vi "LV4_2.vi"() -> ()   [LabVIEW 2011]
uses:
  <vilib>/imath/engines/lvmath2/RunTimeEngine/ErrorHandling/NIMS_Finalize Error.vi
  <vilib>/imath/engines/lvmath2/RunTimeEngine/NodeEndStatement/NIMS_NodeEndStatement_Output.vi
  <instcachedir>/0/NIMS_NodeEndStatement_Output_53EC0D466D134D7ABD903AC30B43404B.lvgen/NIMS_NodeEndStatement_Output_53EC0D466D134D7ABD903AC30B43404B_002.vi
  <instcachedir>/0/NIMS_NodeEndStatement_Output_53EC0D466D134D7ABD903AC30B43404B.lvgen/NIMS_NodeEndStatement_Output_53EC0D466D134D7ABD903AC30B43404B_005.vi
  <instcachedir>/0/NIMS_NodeEndStatement_Output_53EC0D466D134D7ABD903AC30B43404B.lvgen/NIMS_NodeEndStatement_Output_53EC0D466D134D7ABD903AC30B43404B_003.vi
  <vilib>/imath/engines/lvmath2/RunTimeEngine/BuiltInFunctions/linramp/NIMS_linramp.vi
  <vilib>/imath/engines/lvmath2/RunTimeEngine/BuiltInFunctions/residue/NIMS_residue_To Partial Fraction Expansion.vi
  <vilib>/imath/engines/lvmath2/RunTimeEngine/ErrorHandling/NIMS_Error From Error Code.vi
  <vilib>/imath/engines/lvmath2/RunTimeEngine/ArithmeticOperatorToken/NIMS_ArithmeticOperator_multmx.vi
  <instcachedir>/0/NIMS_ArithmeticOperator_multmx_7C179C1E3F6A47AEB223A71AB1A54D0B.lvgen/NIMS_ArithmeticOperator_multmx_7C179C1E3F6A47AEB223A71AB1A54D0B_006.vi
  <vilib>/imath/engines/lvmath2/RunTimeEngine/ArithmeticOperatorToken/NIMS_ArithmeticOperator_multmx(RV,M).vi
  <instcachedir>/0/NIMS_ArithmeticOperator_multmx(RV,M)_0F69384DF375434AAFCFC7849B80E797.lvgen/NIMS_ArithmeticOperator_multmx(RV,M)_0F69384DF375434AAFCFC7849B80E797_000.vi
  <vilib>/imath/engines/lvmath2/RunTimeEngine/ErrorHandling/NIMS_Create Error From Enums.vi
  <vilib>/imath/engines/lvmath2/RunTimeEngine/VariableToken/Read/NIMS_Get Elements - CV(_) - Check.vi
  <instcachedir>/0/NIMS_Get Elements - CV(_) - Check_4CF014B95B49446692066C44E7C19A08.lvgen/NIMS_Get Elements - CV(_) - Check_4CF014B95B49446692066C44E7C19A08_001.vi
  <vilib>/imath/engines/lvmath2/RunTimeEngine/ArithmeticOperatorToken/NIMS_ArithmeticOperator_times.vi
  <instcachedir>/0/NIMS_ArithmeticOperator_times_3FA9DDB491BD45F6905798C0465C9825.lvgen/NIMS_ArithmeticOperator_times_3FA9DDB491BD45F6905798C0465C9825_003.vi
  <vilib>/imath/engines/lvmath2/RunTimeEngine/ArithmeticOperatorToken/NIMS_ArithmeticOperator_plus.vi
  <instcachedir>/0/NIMS_ArithmeticOperator_plus_1E95F7DAB906458CBECCADBE8E6FD739.lvgen/NIMS_ArithmeticOperator_plus_1E95F7DAB906458CBECCADBE8E6FD739_001.vi
  <vilib>/imath/engines/lvmath2/RunTimeEngine/BuiltInFunctions/conv/NIMS_conv(V,V).vi
  <instcachedir>/0/NIMS_conv(V,V)_D3E194F2B5174935BB2368CEB7AAC5A9.lvgen/NIMS_conv(V,V)_D3E194F2B5174935BB2368CEB7AAC5A9_000.vi
  <instcachedir>/0/NIMS_Get Elements - CV(_) - Check_4CF014B95B49446692066C44E7C19A08.lvgen/NIMS_Get Elements - CV(_) - Check_4CF014B95B49446692066C44E7C19A08_002.vi
  <instcachedir>/0/NIMS_ArithmeticOperator_times_3FA9DDB491BD45F6905798C0465C9825.lvgen/NIMS_ArithmeticOperator_times_3FA9DDB491BD45F6905798C0465C9825_008.vi
  <instcachedir>/0/NIMS_ArithmeticOperator_plus_1E95F7DAB906458CBECCADBE8E6FD739.lvgen/NIMS_ArithmeticOperator_plus_1E95F7DAB906458CBECCADBE8E6FD739_009.vi
panel:
  out "Cosine Response":cluster{"t":dbl[], "xstep2":dbl[]}[](graph)
  out "Ramp Response":cluster{"t":dbl[], "xstep2":dbl[]}[](graph)
  out "Step Response":cluster{"t":dbl[], "xstep2":dbl[]}[](graph)
  in  "Period":dbl(slide)=1.0 scale=0.5..5.0
  in  "K2":dbl(slide)=2.0 scale=0.0..10.0
  in  "K1":dbl(slide)=1.25 scale=0.7..2.0
  in  "stop":bool
  in  "K":dbl(slide)=1.25 scale=0.7..2.0
  # "L = 0.625 cm"
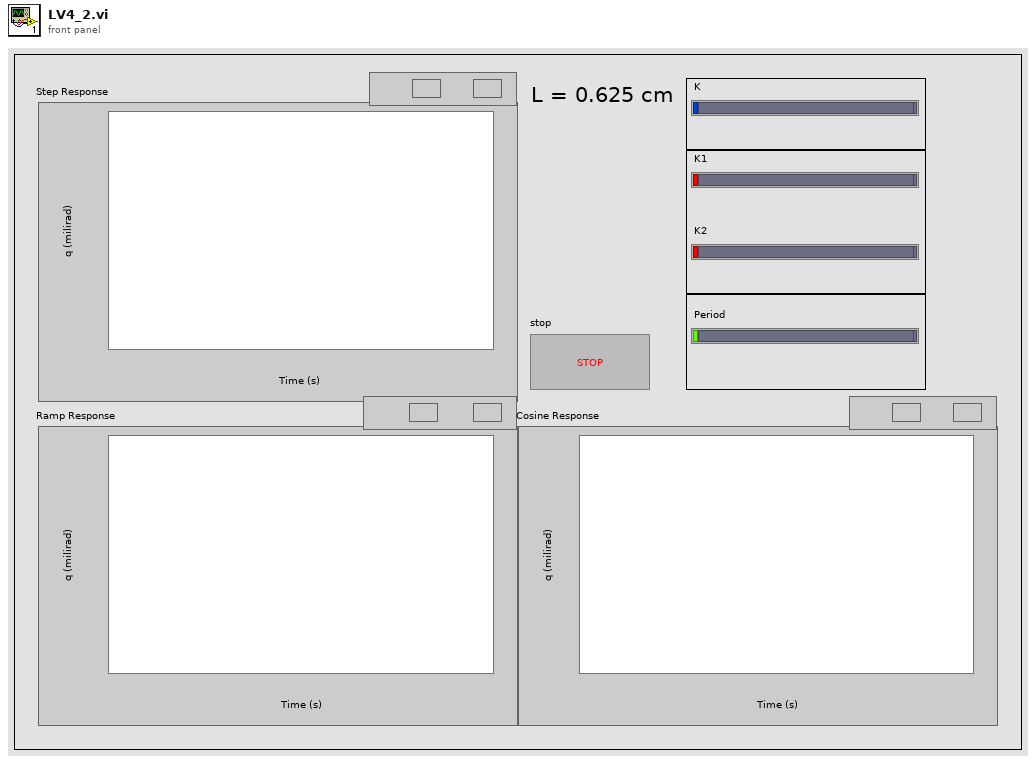
[diagram p1: front panel]
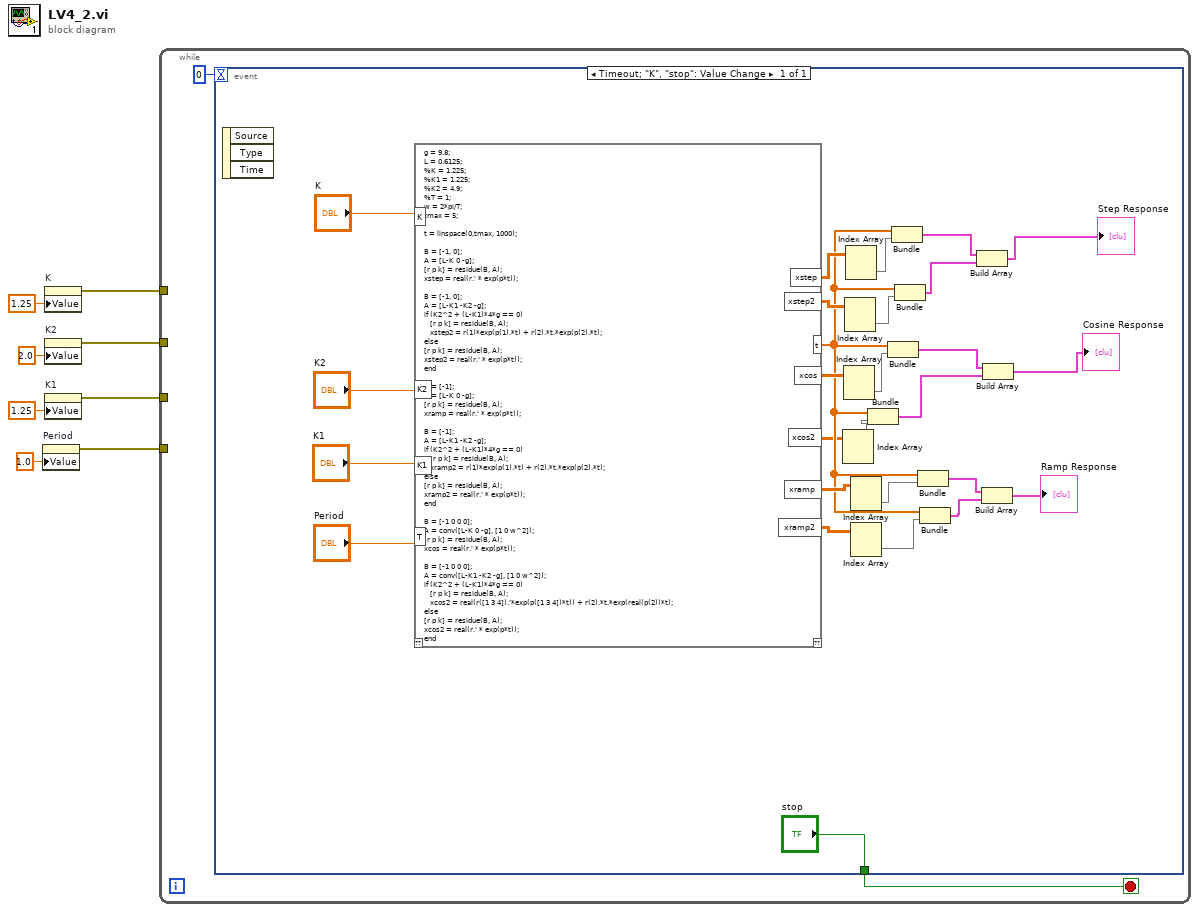
[diagram p0: block diagram]
diagram:
  n1 = property on="Period" class="Slide (strict)"("Value"=1.0 ("Period")) -> (error out=w5:errorcluster)  [unwired: 2 in, 1 out]
  n2 = property on="K" class="Slide (strict)"("Value"=1.25 ("K")) -> (error out=w8:errorcluster)  [unwired: 2 in, 1 out]
  n3 = property on="K2" class="Slide (strict)"("Value"=2.0 ("K2")) -> (error out=w7:errorcluster)  [unwired: 2 in, 1 out]
  n4 = property on="K1" class="Slide (strict)"("Value"=1.25 ("K1")) -> (error out=w6:errorcluster)  [unwired: 2 in, 1 out]
  n5 = while {
    tunnel: w8 -> [_]
    tunnel: w7 -> [_]
    tunnel: w6 -> [_]
    tunnel: w5 -> [_]
    stop <- w10 stop-if-true
    n6 = event shown="[0] Timeout;  \"K\", \"stop\": Value Change" {
      selector: _ -> [_]
      dyn-events: _ -> [_]
      timeout: 0 -> [_]
      tunnel: ["stop"] -> w10
      event Timeout; "K", "stop": Value Change {
        n7 = event-data() -> ()  [unwired: 1 in, 3 out]
        n8 = mathscript code="g = 9.8;\nL = 0.6125;\n%K = 1.225;\n%K1 = 1.225;\n%K2 = 4.9;\n%T = 1;\nw = 2*pi/T;\ntmax = 5;\n\nt = linspace(0,tmax, 1000);\n\nB = [-1, 0];\nA = [L-K 0 -g];\n[r p k] = residue(B, A);\nxstep = real(r.' * exp(p*t));\n\nB = [-1, 0];\nA = [L-K1 -K2 -g];\nif (K2^2 + (L-K1)*4*g == 0)\n   [r p k] = residue(B, A);\n   xstep2 = r(1)*exp(p(1).*t) + r(2).*t.*exp(p(2).*t);\nelse\n[r p k] = residue(B, A);\nxstep2 = real(r.' * exp(p*t));\nend\n\nB = [-1];\nA = [L-K 0 -g];\n[r p k] = residue(B, A);\nxramp = real(r.' * exp(p*t));\n\nB = [-1];\nA = [L-K1 -K2 -g];\nif (K2^2 + (L-K1)*4*g == 0)\n   [r p k] = residue(B, A);\n   xramp2 = r(1)*exp(p(1).*t) + r(2).*t.*exp(p(2).*t);\nelse\n[r p k] = residue(B, A);\nxramp2 = real(r.' * exp(p*t));\nend\n\nB = [-1 0 0 0];\nA = conv([L-K 0 -g], [1 0 w^2]);\n[r p k] = residue(B, A);\nxcos = real(r.' * exp(p*t));\n\nB = [-1 0 0 0];\nA = conv([L-K1 -K2 -g], [1 0 w^2]);\nif (K2^2 + (L-K1)*4*g == 0)\n   [r p k] = residue(B, A);\n   xcos2 = real(r([1 3 4]).'*exp(p([1 3 4])*t)) + r(2).*t.*exp(real(p(2))*t);\nelse\n[r p k] = residue(B, A);\nxcos2 = real(r.' * exp(p*t));\nend"("K1"="K1", "K"="K", "K2"="K2", "T"="Period") -> ("t"=w20:dbl[], "xstep2"=w22:cdb[][], "xramp"=w28:dbl[][], "xramp2"=w26:cdb[][], "xcos"=w31:dbl[][], "xstep"=w24:dbl[][], "xcos2"=w15:cdb[][])  [unwired: 1 in, 1 out]
        n9 = Index Array(array=w15) -> (element=w14:cdb[])  [unwired: 2 in]
        n10 = Index Array(array=w31) -> (element=w30:dbl[])  [unwired: 2 in]
        n11 = Index Array(array=w22) -> (element=w21:cdb[])  [unwired: 2 in]
        n12 = Index Array(array=w24) -> (element=w23:dbl[])  [unwired: 2 in]
        n13 = Index Array(array=w28) -> (element=w27:dbl[])  [unwired: 2 in]
        n14 = Index Array(array=w26) -> (element=w25:cdb[])  [unwired: 2 in]
        n15 = Bundle("t"=w20, "xcos2"=w14) -> (w34:cluster{"t":dbl[], "xcos2":cdb[]})  [unwired: 1 in]
        n16 = Bundle("t"=w20, "xcos"=w30) -> (w29:cluster{"t":dbl[], "xcos":dbl[]})  [unwired: 1 in]
        n17 = Bundle("t"=w20, "xstep"=w23) -> (w19:cluster{"t":dbl[], "xstep":dbl[]})  [unwired: 1 in]
        n18 = Bundle("t"=w20, "xstep2"=w21) -> (w18:cluster{"t":dbl[], "xstep2":cdb[]})  [unwired: 1 in]
        n19 = Bundle("t"=w20, "xramp"=w27) -> (w17:cluster{"t":dbl[], "xramp":dbl[]})  [unwired: 1 in]
        n20 = Bundle("t"=w20, "xramp2"=w25) -> (w16:cluster{"t":dbl[], "xramp2":cdb[]})  [unwired: 1 in]
        n21 = Build Array(w19, w18) -> (→"Step Response":cluster{"t":dbl[], "xstep2":cdb[]}[])
        n22 = Build Array(w17, w16) -> (→"Ramp Response":cluster{"t":dbl[], "xramp2":cdb[]}[])
        n23 = Build Array(w29, w34) -> (→"Cosine Response":cluster{"t":dbl[], "xcos2":cdb[]}[])
      }
    }
  }
